vi "时间查询.vi"() -> (0 "时间标识 3":timestamp format="%<%H:%M:%S\n%x>T", 3 "时间标识 4":timestamp format="%<%H:%M:%S\n%x>T")   [LabVIEW 2016]
panel:
  in  "时间标识 2":timestamp format="%<%H:%M:%S\n%x>T"
  in  "时间标识":timestamp format="%<%H:%M:%S\n%x>T"
  # "至"
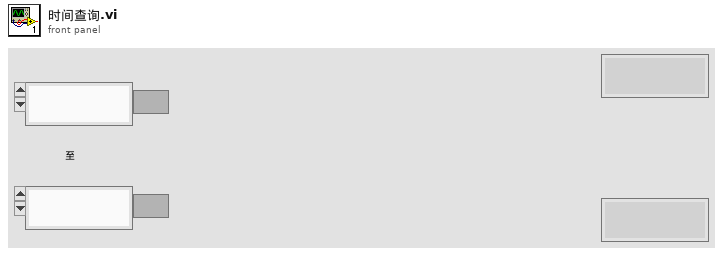
[diagram p1: front panel]
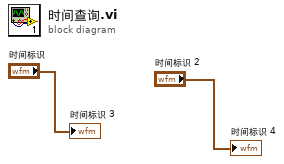
[diagram p0: block diagram]
diagram:
  "时间标识 3" <- "时间标识"
  "时间标识 4" <- "时间标识 2"
